vi "Ctor.vi"(8 "error in (no error)":errorcluster) -> (0 "error out":errorcluster, 3 "TargetPluginManager out":refnum<class "TargetPluginManager.lvclass">)   [LabVIEW 2020, in "PicoG-Core.lvlib" / "TargetPluginManager.lvclass"]
uses:
  TargetPluginManager.lvclass
  Ref Data.ctl
  DeployTarget/DeployTarget.lvclass
  DeployResource/DeployResource.lvclass
  TargetPluginManager.lvclass/TargetPluginManager.ctl
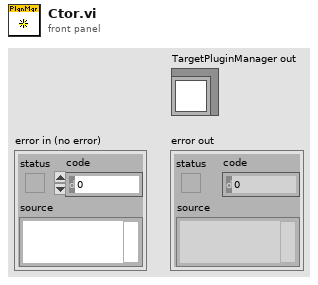
[diagram p1: front panel]
types:
  T1 = typedef "PicoG-Core.lvlib/TargetPluginManager.lvclass/Ref Data.ctl" = cluster{"Targets":refnum<class "DeployTarget.lvclass">[], "Last Target":refnum<class "DeployTarget.lvclass">, "Last Resource":refnum<class "DeployResource.lvclass">}
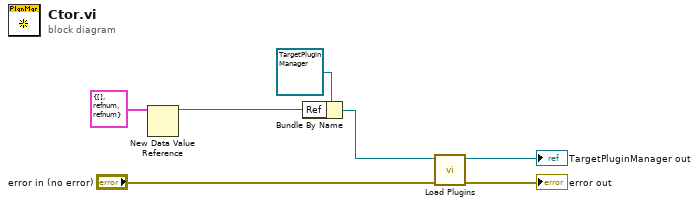
[diagram p0: block diagram]
diagram:
  n1 = New Data Value Reference(data value=T1 {"Targets"=[], "Last Target"=refnum, "Last Resource"=refnum} ("Ref Data")) -> (data value reference=w5:refnum<data-value>)  [unwired: 1 in, 1 out]
  n2 = Bundle By Name(cluster=refnum<class "TargetPluginManager.lvclass"> refnum ("TargetPluginManager in"), "Ref"=w5) -> (w2:refnum<class "TargetPluginManager.lvclass">)
  n3 = call "Load Plugins.vi"("error in (no error)"="error in (no error)", "TargetPluginManager in"=w2) -> ("error out"=→"error out":errorcluster, "TargetPluginManager out"=→"TargetPluginManager out":refnum<class "TargetPluginManager.lvclass">)  [unwired: 8 in]
